vi "Set TCP Listener ref.vi"(10 "Connection ref":refnum<k5>, 11 "TCP Process in":refnum<class "TCP Process.lvclass">) -> (3 "TCP Process out":refnum<class "TCP Process.lvclass">)   [LabVIEW 2019, in "TimingDRV Engine.lvlib" / "TCP Process.lvclass"]
uses:
  TCP Process.lvclass
  TCP Process.lvclass/TCP Process.ctl
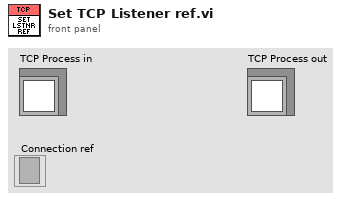
[diagram p1: front panel]
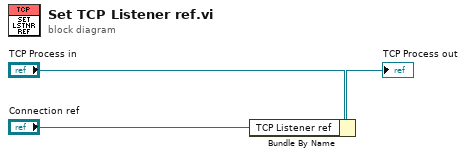
[diagram p0: block diagram]
diagram:
  n1 = Bundle By Name(cluster="TCP Process in", "TCP Listener ref"="Connection ref") -> (→"TCP Process out":refnum<class "TCP Process.lvclass">)
